vi "Apply DSF Configuration to Node.vi"(8 "error in (no error)":errorcluster, 10 "NewVal":path, 11 "Item Ref in":T2 format="%.0x") -> (0 "error out":errorcluster, 3 "version":T1)   [LabVIEW 2017, in "DSF System Explorer.lvlib"]
uses:
  DSF System Explorer.lvlib
  <vilib>/NI Veristand/Custom Device API/Custom Device Item Ref.ctl
  DSF Core.lvlibp/Typedefs/DSF Version Info.ctl
  <vilib>/NI Veristand/Custom Device API/Custom Device API.lvlib
  DSF Core.lvlibp
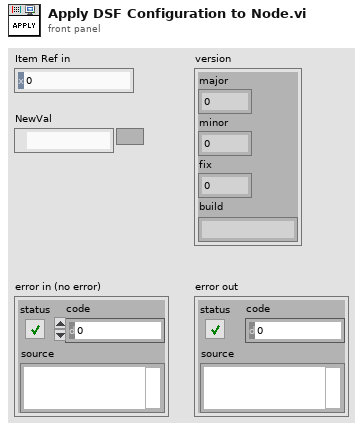
[diagram p1: front panel]
types:
  T1 = typedef "DSF Core.lvlibp/DSF Version Info.ctl" = cluster{"major":u32, "minor":u32, "fix":u32, "build":string}
  T2 = typedef "Custom Device API.lvlib/Custom Device Item Ref.ctl" = u64
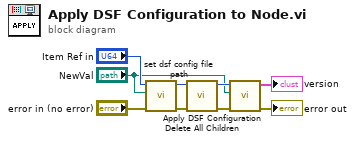
[diagram p0: block diagram]
diagram:
  n1 = call "set dsf config file path.vi"("error in (no error)"="error in (no error)", "Path"="NewVal", "Item Ref in"="Item Ref in") -> ("error out"=w3:errorcluster, "Item Ref out"=w4:T2)  [unwired: 7 in]
  n2 = call "Delete All Children.vi"("error in (no error)"=w3, "Item Ref in"=w4) -> ("error out"=w8:errorcluster, "Item Ref out"=w9:T2)  [unwired: 8 in]
  n3 = call "Apply DSF Configuration.vi"("error in (no error)"=w8, "config path"="NewVal", "Item Ref in"=w9) -> ("error out"=→"error out":errorcluster, "version"=→"version":T1)  [unwired: 7 in]
